vi "get wavefront array from slopes.vi"(8 "error in (no error)":errorcluster, 11 "HasoSlopes in":refnum<class "HasoSlopes.lvclass">) -> (0 "error out":errorcluster, 2 "data":sgl[][](array[numeric]), 3 "StatisticsData":T1)   [LabVIEW 2020, in "HASO4_3.lvclass"]
uses:
  HASO4_3.lvclass
  WaveKit/Classes/HasoSlopes/HasoSlopes.lvclass
  WaveKit/Controls/StatisticsData.ctl
  WaveKit/Classes/Phase/Phase.lvclass
  WaveKit/Classes/Pupil/Pupil.lvclass
  WaveKit/Classes/HasoData/HasoData.lvclass
  WaveKit/Classes/ComputePhaseSet/ComputePhaseSet.lvclass
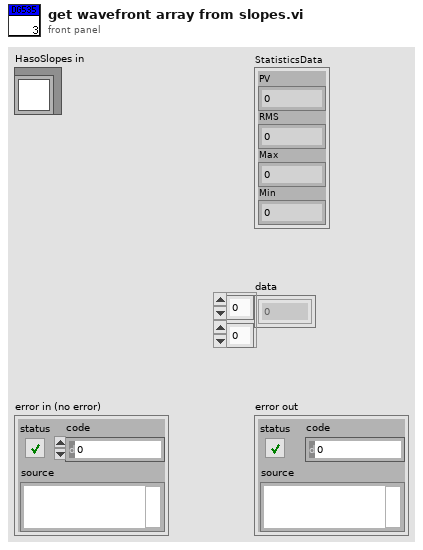
[diagram p1: front panel]
types:
  T1 = typedef "StatisticsData.ctl" = cluster{"PV":sgl, "RMS":dbl, "Max":sgl, "Min":sgl}
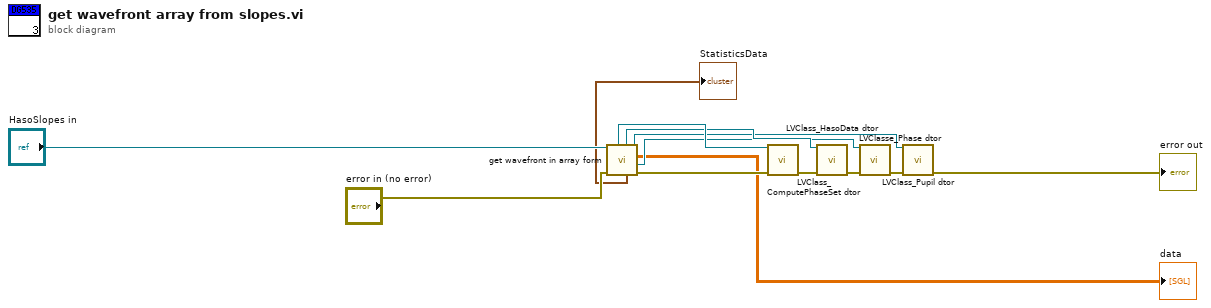
[diagram p0: block diagram]
diagram:
  n1 = call "get wavefront in array form.vi"("error in (no error)"="error in (no error)", "HasoSlopes in"="HasoSlopes in") -> ("error out"=w10:errorcluster, "Phase out"=w3:refnum<class "Phase.lvclass">, "data"=→"data":sgl[][], "Pupil out"=w4:refnum<class "Pupil.lvclass">, "StatisticsData"=→"StatisticsData":T1, "HasoData out"=w7:refnum<class "HasoData.lvclass">, "ComputePhaseSet.lvclass 2"=w8:refnum<class "ComputePhaseSet.lvclass">)  [unwired: 3 in]
  n2 = call "LVClass_ComputePhaseSet dtor.vi"("ComputePhaseSet in"=w8, "error in (no error)"=w10) -> ("error out"=w9:errorcluster)  [unwired: 12 in, 1 out]
  n3 = call "LVClass_HasoData dtor.vi"("HasoData in"=w7, "error in (no error)"=w9) -> ("error out"=w11:errorcluster)  [unwired: 12 in, 1 out]
  n4 = call "LVClasse_Phase dtor.vi"("Phase in"=w3, "error in (no error)"=w11) -> ("error out"=w5:errorcluster)  [unwired: 12 in, 1 out]
  n5 = call "LVClass_Pupil dtor.vi"("Pupil in"=w4, "error in (no error)"=w5) -> ("error out"=→"error out":errorcluster)  [unwired: 12 in, 1 out]
